vi "Persist New Entity.vi"(8 "error in (no error)":errorcluster, 10 "Conditum:Entity":refnum<class "Entity.lvclass">, 11 "SQLite in":refnum<class "SQLite.lvclass">) -> (0 "error out":errorcluster, 2 "Entity ID":T1, 3 "SQLite out":refnum<class "SQLite.lvclass">)   [LabVIEW 2022 SP3, in "Conditum SQLite.lvlib" / "SQLite.lvclass"]
uses:
  SQLite.lvclass
  <vilib>/IlluminatedG/IG Conditum/Conditum/Entity/Entity.lvclass
  <vilib>/IlluminatedG/IG Conditum/Conditum/Entity ID.ctl
  SQLite.lvclass/SQLite.ctl
  <vilib>/IlluminatedG/IG Conditum/Conditum/Entity/Entity.lvclass/Entity.ctl
  <vilib>/IlluminatedG/IG Conditum/Conditum/Columns/Type/Type.lvclass/Type.ctl
  <vilib>/IlluminatedG/IG Conditum/Conditum/Columns/Boolean/Boolean.lvclass
  <vilib>/IlluminatedG/IG Conditum/Conditum/Columns/Boolean/Boolean.lvclass/Boolean.ctl
  <vilib>/drjdpowell/SQLite Library/SQL Statement/SQL Statement.lvclass/SQL Statement.ctl
  <vilib>/IlluminatedG/IG Conditum/Conditum/Columns/Integer/Integer.lvclass
  <vilib>/IlluminatedG/IG Conditum/Conditum/Columns/Integer/Integer.lvclass/Integer.ctl
  <vilib>/IlluminatedG/IG Conditum/Conditum/Columns/Double/Double.lvclass
  <vilib>/IlluminatedG/IG Conditum/Conditum/Columns/Timestamp/Timestamp.lvclass
  <vilib>/IlluminatedG/IG Conditum/Conditum/Columns/Timestamp/Timestamp.lvclass/Timestamp.ctl
  <vilib>/IlluminatedG/IG Conditum/Conditum/Columns/String/String.lvclass
  <vilib>/IlluminatedG/IG Conditum/Conditum/Columns/String/String.lvclass/String.ctl
  <vilib>/drjdpowell/SQLite Library/SQL Connection/Connection.lvclass/Connection.ctl
  <vilib>/drjdpowell/SQLite Library/SQL Statement/Bind Integer.vi
  <vilib>/drjdpowell/SQLite Library/SQL Statement/Bind Real.vi
  <vilib>/drjdpowell/SQLite Library/SQL Statement/Bind Timestamp (Text).vi
  <vilib>/drjdpowell/SQLite Library/SQL Statement/Bind Text.vi
  <vilib>/JDP Science/JDP Science Common Utilities/Timestamp/Timestamp to Text.vi
  <vilib>/drjdpowell/SQLite Library/SQL Statement/Step.vi
  <vilib>/IlluminatedG/IG Conditum/Conditum/Columns/ID/ID.lvclass
  C:/Program Files (x86)/National Instruments/LabVIEW 2022/vi.lib/IlluminatedG/IG Conditum/Conditum/Columns/Type/Type.lvclass
  <vilib>/drjdpowell/SQLite Library/SQL Statement/Error Message.vi
  <vilib>/drjdpowell/SQLite Library/SQL Connection/Connection.lvclass
  <vilib>/drjdpowell/SQLite Library/Transaction Helpers/Transaction.lvlib
  <vilib>/IlluminatedG/IG Conditum/Conditum/Columns/Type/Type.lvclass
  <vilib>/drjdpowell/SQLite Library/SQL Statement/SQL Statement.lvclass
  <vilib>/IlluminatedG/IG Conditum/Conditum/Conditum.lvlib
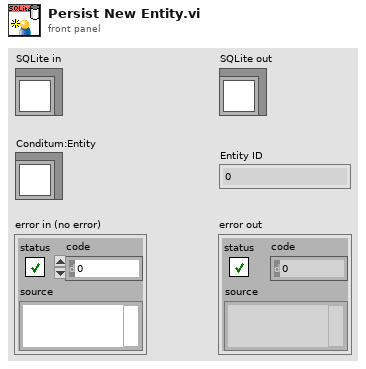
[diagram p1: front panel]
types:
  T1 = typedef "Conditum.lvlib/Entity ID.ctl" = i64
  T2 = typedef "Conditum.lvlib/LabVIEW Type.ctl" = enum16{"None", "ID", "Boolean", "Integer", "Double", "Timestamp", "String", "Text", "Entity"}
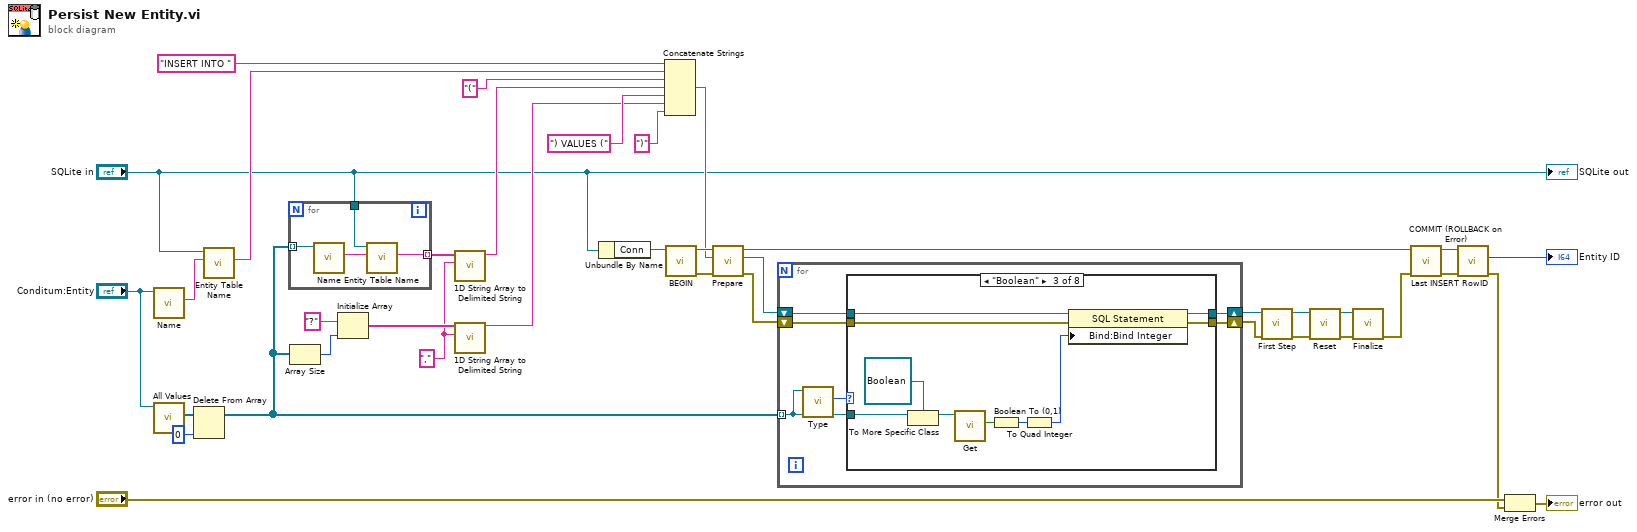
[diagram p0: block diagram]
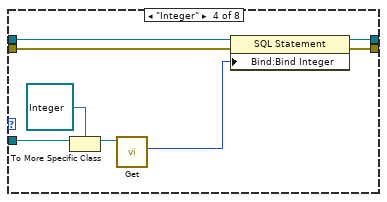
[diagram p4: hidden frame]
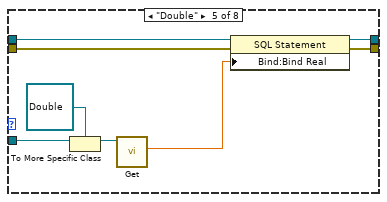
[diagram p5: hidden frame]
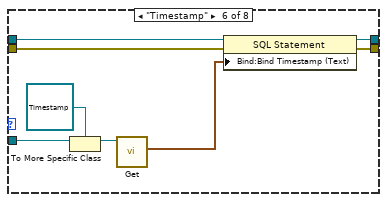
[diagram p6: hidden frame]
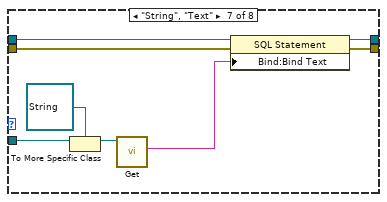
[diagram p7: hidden frame]
diagram:
  w4 = "," ("delimiter")
  n1 = call-dynamic <vilib>:"Name.vi"("Entity in"="Conditum:Entity") -> ("Name"=w37:string)  [unwired: 10 in]
  n2 = call <vilib>:"All Values.vi"("Entity in"="Conditum:Entity") -> ("All Values"=w36:refnum<class "Type.lvclass">[])  [unwired: 10 in]
  n3 = Delete From Array(array=w36, index=0) -> (array with subset deleted=w6:refnum<class "Type.lvclass">[])  [unwired: 1 in, 1 out]
  n4 = call-dynamic "Entity Table Name.vi"("Entity Name"=w37, "Database in"="SQLite in") -> ("Table Name"=w32:string)  [unwired: 9 in]
  n5 = for {
    tunnel: w6 -> [w42] mode=indexing
    tunnel: [w40] -> w5 mode=indexing
    tunnel: "SQLite in" -> [w39]
    n6 = call <vilib>:"Name.vi"("Type in"=w42) -> ("Table Name"=w41:string)  [unwired: 10 in]
    n7 = call-dynamic "Entity Table Name.vi"("Entity Name"=w41, "Database in"=w39) -> ("Table Name"=w40:string)  [unwired: 9 in]
  }
  n8 = Array Size(array=w6) -> (size(s)=w31:i32)
  n9 = Initialize Array("?", w31) -> (w29:string[])
  n10 = call <vilib>:"1D String Array to Delimited String.vi"("delimiter"=w4, "string array"=w5) -> ("delimited string"=w2:string)  [unwired: 9 in]
  n11 = call <vilib>:"1D String Array to Delimited String.vi"("delimiter"=w4, "string array"=w29) -> ("delimited string"=w27:string)  [unwired: 9 in]
  n12 = Unbundle By Name("SQLite in") -> ("Conn"=w25:refnum<class "Connection.lvclass">)
  n13 = Concatenate Strings("INSERT INTO ", w32, "(" ("string"), w2, ") VALUES (" ("string"), w27, ")" ("string")) -> (w22:string)
  n14 = call <vilib>:"BEGIN.vi"("SQLite Connection in"=w25) -> ("error out"=w23:errorcluster, "SQLite Connection"=w24:refnum<class "Connection.lvclass">)  [unwired: 9 in]
  n15 = call <vilib>:"Prepare.vi"("error in (no error)"=w23, "SQL"=w22, "SQLite Connection in"=w24) -> ("error out"=w20:errorcluster, "SQL Statement"=w21:refnum<class "SQL Statement.lvclass">, "SQLite Connection"=w13:refnum<class "Connection.lvclass">)  [unwired: 4 in, 2 out]
  n16 = for {
    shift-right: [w44] -> w19
    shift-left: w21 -> [w48]
    shift-right: [w43] -> w18
    shift-left: w20 -> [w47]
    tunnel: w6 -> [w45] mode=indexing
    n17 = call <vilib>:"Type.vi"("Type in"=w45) -> ("Type"=w46:T2)  [unwired: 10 in]
    n18 = case shown="\"Boolean\"" w46 {
      tunnel: w48 -> [w50 w52 w59 w67 w75 w83 w91 w96]
      tunnel: w47 -> [w49 w51 w55 w66 w74 w82 w90 w95]
      tunnel: w45 -> [_ _ w62 w70 w78 w86 w94 _]
      tunnel: [w50 w52 w54 w65 w73 w81 w89 w96] -> w44
      tunnel: [w49 w51 w53 w64 w72 w80 w88 w95] -> w43
      frame "None", Default {
        # "#ERROR"
      }
      frame "ID" {
        # "#ERROR"
      }
      frame "Boolean" {
        n19 = To More Specific Class(target class=refnum<class "Boolean.lvclass"> refnum ("Conditum:Columns:Boolean.lvclass"), reference=w62) -> (specific class reference=w60:refnum<class "Boolean.lvclass">)  [unwired: 1 in, 1 out]
        n20 = call <vilib>:"Get.vi"("Boolean in"=w60) -> ("Value"=w58:bool)  [unwired: 10 in]
        n21 = Boolean To (0,1)(Boolean=w58) -> (0, 1=w57:i16)
        n22 = To Quad Integer(1:w57) -> (0:w56:i64)
        n23 = property class="SQL Statement"(reference=w59, error in=w55, "Bind:Bind Integer"=w56) -> (reference out=w54:refnum<class "SQL Statement.lvclass">, error out=w53:errorcluster)
      }
      frame "Integer" {
        n24 = To More Specific Class(target class=refnum<class "Integer.lvclass"> refnum ("Conditum:Columns:Integer.lvclass"), reference=w70) -> (specific class reference=w68:refnum<class "Integer.lvclass">)  [unwired: 1 in, 1 out]
        n25 = call <vilib>:"Get.vi"("Integer in"=w68) -> ("Value"=w63:i64)  [unwired: 10 in]
        n26 = property class="SQL Statement"(reference=w67, error in=w66, "Bind:Bind Integer"=w63) -> (reference out=w65:refnum<class "SQL Statement.lvclass">, error out=w64:errorcluster)
      }
      frame "Double" {
        n27 = To More Specific Class(target class=refnum<class "Double.lvclass"> refnum ("Conditum:Columns:Double.lvclass"), reference=w78) -> (specific class reference=w76:refnum<class "Double.lvclass">)  [unwired: 1 in, 1 out]
        n28 = call <vilib>:"Get.vi"("Double in"=w76) -> ("Value"=w71:dbl)  [unwired: 10 in]
        n29 = property class="SQL Statement"(reference=w75, error in=w74, "Bind:Bind Real"=w71) -> (reference out=w73:refnum<class "SQL Statement.lvclass">, error out=w72:errorcluster)
      }
      frame "Timestamp" {
        n30 = To More Specific Class(target class=refnum<class "Timestamp.lvclass"> refnum ("Conditum:Columns:Timestamp.lvclass"), reference=w86) -> (specific class reference=w84:refnum<class "Timestamp.lvclass">)  [unwired: 1 in, 1 out]
        n31 = call <vilib>:"Get.vi"("Timestamp in"=w84) -> ("Value"=w79:timestamp)  [unwired: 10 in]
        n32 = property class="SQL Statement"(reference=w83, error in=w82, "Bind:Bind Timestamp (Text)"=w79) -> (reference out=w81:refnum<class "SQL Statement.lvclass">, error out=w80:errorcluster)
      }
      frame "String", "Text" {
        n33 = To More Specific Class(target class=refnum<class "String.lvclass"> refnum ("Conditum:Columns:String.lvclass"), reference=w94) -> (specific class reference=w92:refnum<class "String.lvclass">)  [unwired: 1 in, 1 out]
        n34 = call <vilib>:"Get.vi"("String in"=w92) -> ("Value"=w87:string)  [unwired: 10 in]
        n35 = property class="SQL Statement"(reference=w91, error in=w90, "Bind:Bind Text"=w87) -> (reference out=w89:refnum<class "SQL Statement.lvclass">, error out=w88:errorcluster)
      }
      frame "Entity" {
        # "#TODO\nRelation update"
      }
    }
  }
  n36 = call <vilib>:"First Step.vi"("error in (no error)"=w18, "SQL Statement in"=w19) -> ("error out"=w17:errorcluster, "SQL Statement"=w16:refnum<class "SQL Statement.lvclass">)  [unwired: 7 in, 1 out]
  n37 = call <vilib>:"Reset.vi"("error in (no error)"=w17, "SQL Statement in"=w16) -> ("error out"=w15:errorcluster, "SQL Statement"=w14:refnum<class "SQL Statement.lvclass">)  [unwired: 8 in]
  n38 = call <vilib>:"Finalize.vi"("error in (no error)"=w15, "SQL Statement in"=w14) -> ("error out"=w10:errorcluster)  [unwired: 9 in]
  n39 = call <vilib>:"COMMIT (ROLLBACK on Error).vi"("error in (no error)"=w10, "SQLite Connection in"=w13) -> ("error out"=w12:errorcluster, "SQLite Connection"=w11:refnum<class "Connection.lvclass">)  [unwired: 8 in]
  n40 = call <vilib>:"Last INSERT RowID.vi"("error in (no error)"=w12, "SQLite Connection in"=w11) -> ("error out"=w7:errorcluster, "Last INSERT RowID"=→"Entity ID":i64)  [unwired: 7 in, 1 out]
  n41 = Merge Errors("error in (no error)", w7) -> (→"error out":errorcluster)
  "SQLite out" <- "SQLite in"
